vi "DumbDash Control Filter.vi"(11 "Ctl Refnum":refnum<vi>) -> (2 "Keep?":bool)   [LabVIEW 2014]
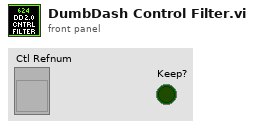
[diagram p1: front panel]
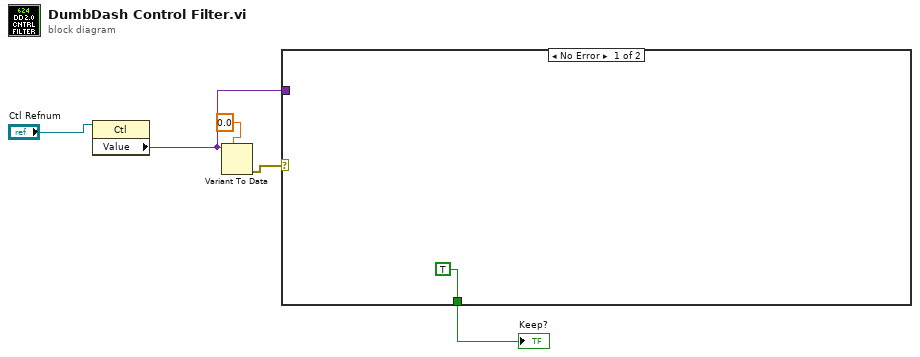
[diagram p0: block diagram]
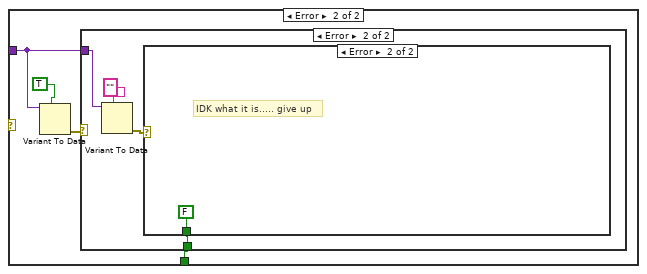
[diagram p2: hidden frame]
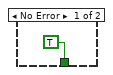
[diagram p3: hidden frame]
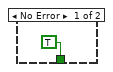
[diagram p4: hidden frame]
diagram:
  n1 = property class="Ctl"(reference="Ctl Refnum") -> ("Value"=w2:variant)  [unwired: 1 in, 2 out]
  n2 = Variant To Data(type=0.0, Variant=w2) -> (error out=w3:errorcluster)  [unwired: 1 in, 1 out]
  n3 = case shown="No Error" w3 {
    tunnel: w2 -> [_ w8]
    tunnel: [TRUE w7] -> w1
    frame No Error {
    }
    frame Error {
      n4 = Variant To Data(type=TRUE, Variant=w8) -> (error out=w9:errorcluster)  [unwired: 1 in, 1 out]
      n5 = case shown="Error" w9 {
        tunnel: w8 -> [_ w15]
        tunnel: [TRUE w12] -> w7
        frame No Error {
        }
        frame Error {
          n6 = Variant To Data(type="", Variant=w15) -> (error out=w13:errorcluster)  [unwired: 1 in, 1 out]
          n7 = case shown="Error" w13 {
            tunnel: [TRUE FALSE] -> w12
            frame No Error {
            }
            frame Error {
              # "IDK what it is..... give up"
            }
          }
        }
      }
    }
  }
  "Keep?" <- w1
